vi "StartDebugServer.vi"(1 "TCP port":u16=62001, 5 "error in (no error)":errorcluster) -> (19 "error out":errorcluster)   [LabVIEW 2017, in "G#DebugServer.lvclass"]
doc: "Starts the debug server process that makes it possible for the G# Debugger on the client host to debug objects on this remote target. Garbage collector will stop this debug process."
uses:
  G#DebugServer.lvclass
  G#Object/G#Object.lvclass
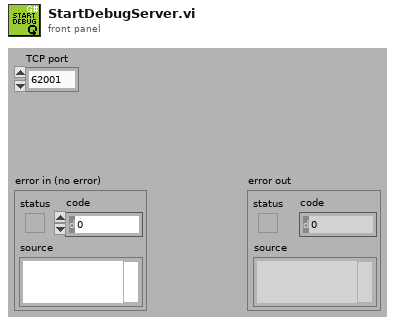
[diagram p1: front panel]
types:
  T1 = enum32{"Bad", "Idle", "Run top level", "Running"}
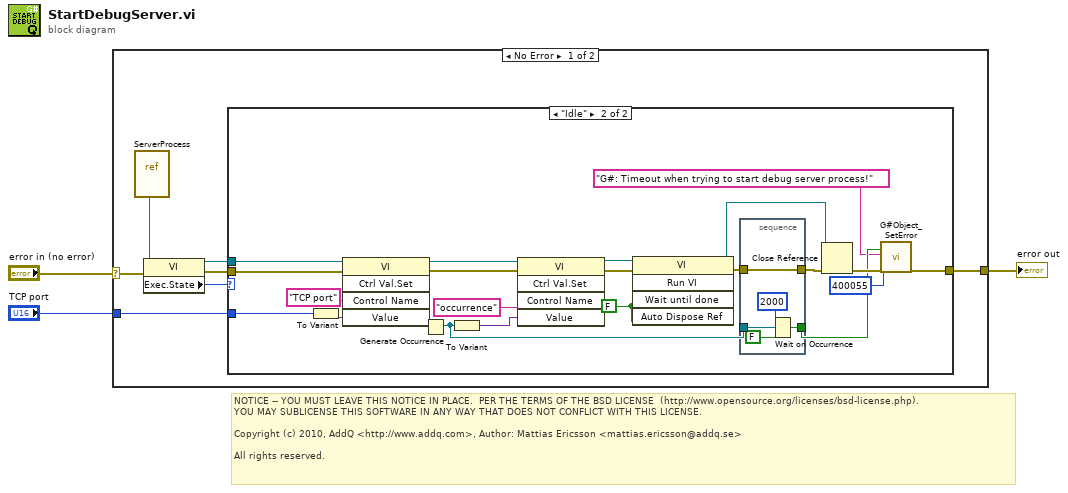
[diagram p0: block diagram]
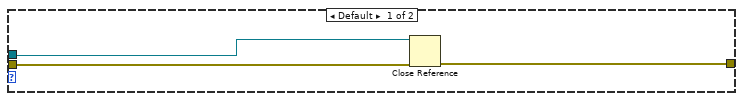
[diagram p2: hidden frame]
diagram:
  # "NOTICE -- YOU MUST LEAVE THIS NOTICE IN PLACE.  PER THE TERMS OF THE BSD LICENSE  (http://www.opensource.org/licenses/bsd-license.php).\nYOU MAY SUBLICENSE THIS SOFTWARE IN ANY WAY THAT DOES NOT CONFLICT WITH THIS LICENSE.\n\nCopyright (c) 2010, AddQ <http://www.addq.com>, Author: Mattias Ericsson <mattias.ericsson@addq.se>\n\nAll rights reserved."
  n1 = case shown="No Error" "error in (no error)" {
    selector: "error in (no error)" -> [w5 w40]
    tunnel: [w6 w40] -> w2
    tunnel: "TCP port" -> [w4 _]
    frame No Error {
      n2 = vi-ref "ServerProcess.vi"() -> (w10:refnum<vi>)
      n3 = property class="VI"(reference=w10, error in=w5) -> (reference out=w7:refnum<vi>, error out=w8:errorcluster, "Exec.State"=w9:T1)
      n4 = case shown="\"Idle\"" w9 {
        tunnel: w8 -> [w13 w18]
        tunnel: w7 -> [w11 w17]
        tunnel: [w12 w24] -> w6
        tunnel: w4 -> [_ w15]
        frame Default {
          n5 = Close Reference(reference=w11, error in (no error)=w13) -> (error out=w12:errorcluster)
        }
        frame "Idle" {
          w30 = FALSE ("Wait Until Done")
          n6 = To Variant(anything=w15) -> (Variant=w16:variant)
          n7 = invoke class="VI" method="Ctrl Val.Set"(reference=w17, error in=w18, "Control Name"="TCP port", "Value"=w16) -> (reference out=w19:refnum<vi>, error out=w20:errorcluster)  [unwired: 1 in, 3 out]
          n8 = Generate Occurrence() -> (w28:refnum<k4>)
          n9 = To Variant(anything=w28) -> (Variant=w33:variant)
          n10 = invoke class="VI" method="Ctrl Val.Set"(reference=w19, error in=w20, "Control Name"="occurrence", "Value"=w33) -> (reference out=w31:refnum<vi>, error out=w32:errorcluster)  [unwired: 1 in, 3 out]
          n11 = invoke class="VI" method="Run VI"(reference=w31, error in=w32, "Wait until done"=w30, "Auto Dispose Ref"=w30) -> (reference out=w26:refnum<vi>, error out=w29:errorcluster)  [unwired: 1 in, 3 out]
          n12 = stacked-sequence {
            tunnel: w29 -> [w37]
            tunnel: w28 -> [w39]
            tunnel: [w37] -> w27
            tunnel: [w36] -> w23
            frame #0 {
              n13 = Wait on Occurrence(1:FALSE ("ignore previous (T)"), 2:w39, 3:2000 ("ms timeout (-1)")) -> (0:w36:bool)
            }
          }
          n14 = Close Reference(reference=w26, error in (no error)=w27) -> (error out=w25:errorcluster)
          n15 = call "G#Object_SetError.vi"("error (F)"=w23, "source"="G#: Timeout when trying to start debug server process!", "code"=400055, "error in (no error)"=w25) -> ("error out"=w24:errorcluster)  [unwired: 15 in]
        }
      }
    }
    frame Error {
    }
  }
  "error out" <- w2
